vi "IOTest Target.vi"() -> ()   [LabVIEW 2012]
uses:
  <vilib>/rvi/FXPMathLib/basic elements/FxpIntAccumulator/subVIs/nifxpmath_IntAccumulator_SimConfig.ctl
  <vilib>/rvi/FXPMathLib/FxpSinAndCos/subVIs/nifxpmath_SinAndCos_SimConfig.ctl
  <vilib>/rvi/FXPMathLib/basic elements/FxpIntAccumulator/simVIs/DllFxpIntAccumulator_sub.vi
  <vilib>/rvi/FXPMathLib/FxpSinAndCos/simVIs/DllFxpSinAndCosTemp_sub.vi
  <vilib>/rvi/eio/common/nirviEmuTemplateMethod_errors.vi
  <vilib>/rvi/FXPMathLib/basic elements/FxpIntAccumulator/XNode/nifxpmath_IntAccumulator.xnode
  <vilib>/rvi/FXPMathLib/FxpSinAndCos/XNode/nifxpmath_SinAndCos.xnode
  <vilib>/eio/EIONode/EIONode.xnode
panel:
  out "Signal Graph":i16(graph)
  in  "Load":bool
  in  "Frequency":i16
  in  "Start":bool
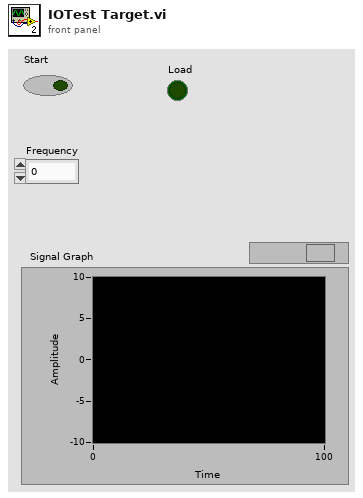
[diagram p1: front panel]
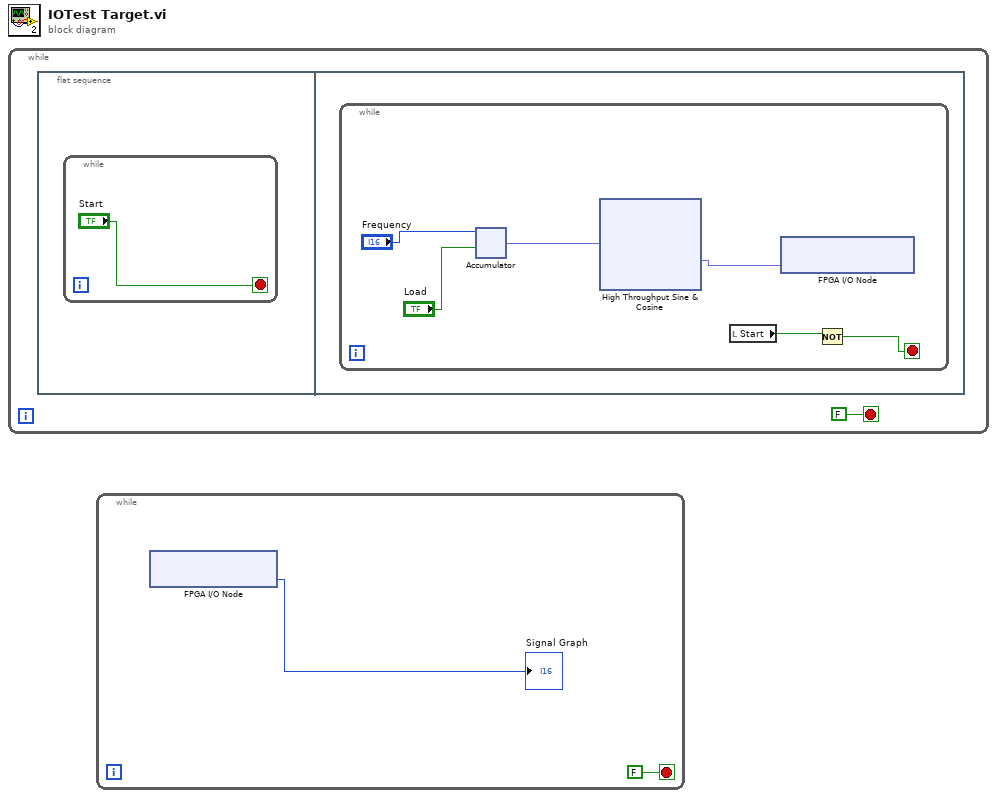
[diagram p0: block diagram]
diagram:
  n1 = while {
    stop <- FALSE stop-if-true
    n2 = flat-sequence {
      frame #0 {
        n3 = while {
          stop <- "Start" stop-if-true
        }
      }
      frame #1 {
        n4 = while {
          stop <- w7 stop-if-true
          n5 = xnode "Accumulator"("x"="Frequency", "load (F)"="Load") -> ("s"=w5:fxp<+/-,32,32>)  [unwired: 3 in, 1 out]
          n6 = xnode "High Throughput Sine & Cosine"("x (pi)"=w5) -> ("sin(x)"=w4:fxp<+/-,16,2>)  [unwired: 1 out]
          n7 = local read "Start"() -> (w8:bool)
          n8 = xnode "FPGA I/O Node"("Connector0/AO1"=w4) -> ()  [unwired: 1 in, 1 out]
          n9 = Not(x=w8) -> (.not. x?=w7:bool)
        }
      }
    }
  }
  n10 = while {
    stop <- FALSE stop-if-true
    n11 = xnode "FPGA I/O Node"() -> ("Connector0/AI3"=→"Signal Graph":i16)  [unwired: 1 in, 1 out]
  }
